vi "find_terms_by_names.vi"(9 "Name":string, 10 "Terminals[]":refnum<vi>[](array[refnum])) -> (2 "reference out":refnum<vi>)   [LabVIEW 2018]
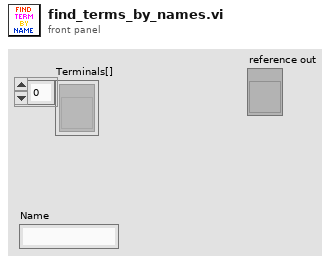
[diagram p1: front panel]
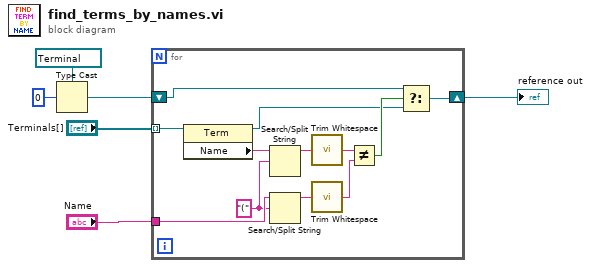
[diagram p0: block diagram]
diagram:
  n1 = Type Cast(type=refnum<vi> refnum ("Term"), x=0) -> (*(type *) &x=w2:refnum<vi>)
  n2 = for {
    tunnel: "Terminals[]" -> [w18] mode=indexing
    tunnel: "Name" -> [w14]
    shift-right: [w7] -> w1
    shift-left: w2 -> [w9]
    w13 = "(" ("search string/char (-)")
    n3 = property class="Term"(reference=w18) -> (reference out=w8:refnum<vi>, "Name"=w17:string)  [unwired: 1 in, 1 out]
    n4 = Search/Split String(string=w17, search string/char (-)=w13) -> (substring before match=w16:string)  [unwired: 1 in, 2 out]
    n5 = Search/Split String(string=w14, search string/char (-)=w13) -> (substring before match=w12:string)  [unwired: 1 in, 2 out]
    n6 = call <vilib>:"Trim Whitespace.vi"("string"=w16) -> ("trimmed string"=w15:string)  [unwired: 1 in]
    n7 = call <vilib>:"Trim Whitespace.vi"("string"=w12) -> ("trimmed string"=w11:string)  [unwired: 1 in]
    n8 = Not Equal?(x=w15, y=w11) -> (x != y?=w10:bool)
    n9 = Select(t=w9, s=w10, f=w8) -> (s? t:f=w7:refnum<vi>)
  }
  "reference out" <- w1
